vi "读取文件路径.vi"(8 "error in (no error)":errorcluster caption="错误输入（无错误）", 11 "程序输入":refnum<class "程序.lvclass">) -> (0 "error out":errorcluster caption="错误输出", 2 "文件路径":path, 3 "程序输出":refnum<class "程序.lvclass">)   [LabVIEW 2020, in "程序.lvclass"]
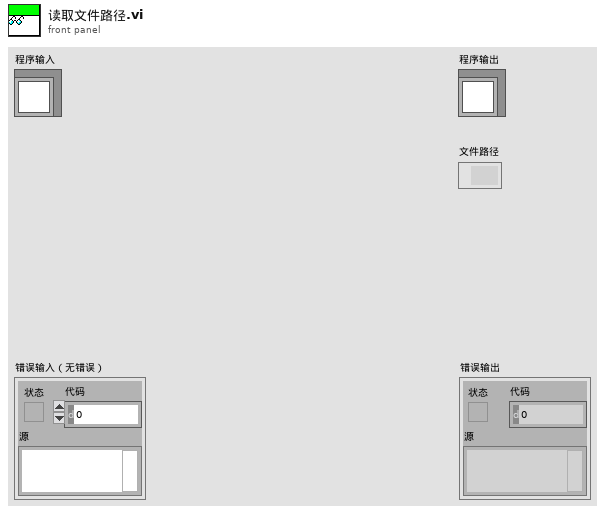
[diagram p1: front panel]
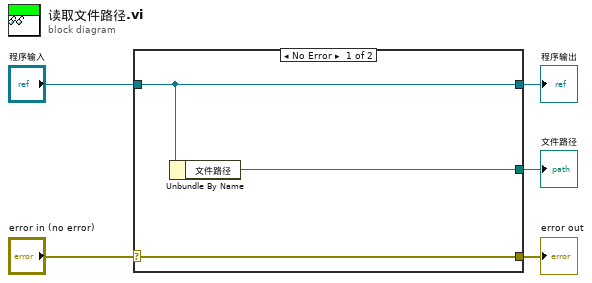
[diagram p0: block diagram]
diagram:
  n1 = case shown="No Error" "error in (no error)" {
    selector: "error in (no error)" -> [w8 w9]
    tunnel: [w8 w9] -> w4
    tunnel: [w7 w10] -> w2
    tunnel: "程序输入" -> [w7 w10]
    tunnel: [w6 _] -> w1
    frame No Error {
      n2 = Unbundle By Name(w7) -> ("文件路径"=w6:path)
    }
    frame Error {
    }
  }
  "error out" <- w4
  "程序输出" <- w2
  "文件路径" <- w1
